vi "find_correction.vi"(9 "T1_parameters":T1, 10 "triggers":u32[][](array[numeric]), 11 "detections":u32[](array[numeric])) -> (3 "shift_us":dbl)   [LabVIEW 2014]
uses:
  <vilib>/Analysis/3filter.llb/FIR Filter (DBL).vi
  <vilib>/Analysis/NI_AALPro.lvlib
  <vilib>/Analysis/NI_AALBase.lvlib
panel:
  out "pulses":u32[](graph)
  out "derivative":dbl[](graph)
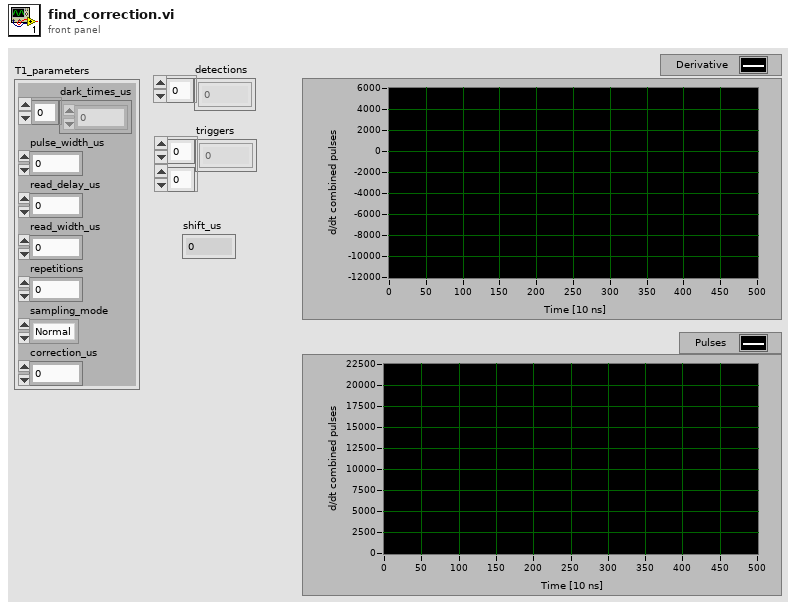
[diagram p1: front panel]
types:
  T1 = cluster{"dark_times_us":dbl[], "pulse_width_us":dbl, "read_delay_us":dbl, "read_width_us":dbl, "repetitions":i32, "sampling_mode":enum16{"Normal", "Sweep"}, "correction_us":dbl}
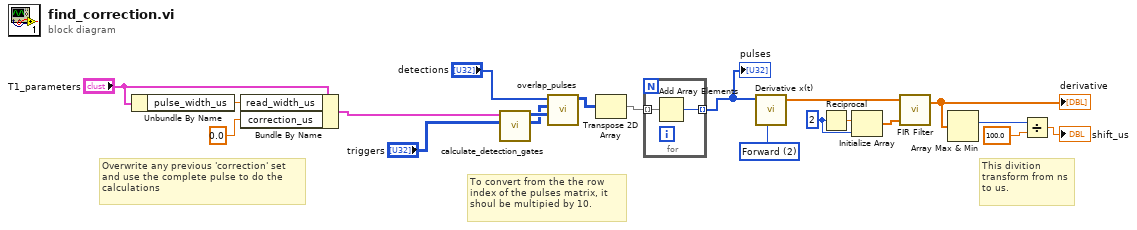
[diagram p0: block diagram]
diagram:
  w4 = 2 ("dimension size")
  w19 = u16 2 items=["2nd Order Central", "4th Order Central", "Forward", "Backward"] ("method")
  # "Overwrite any previous 'correction' set\nand use the complete pulse to do the\ncalculations"
  # "This divition transform from ns to us."
  # "To convert from the the row index of the pulses matrix, it shoul be multipied by 10."
  n1 = Unbundle By Name("T1_parameters") -> ("pulse_width_us"=w15:dbl)
  n2 = Bundle By Name(cluster="T1_parameters", "read_width_us"=w15, "correction_us"=0.0) -> (w7:T1)
  n3 = call "calculate_detection_gates.vi"("triggers"="triggers", "T1_parameters"=w7) -> ("start_read"=w11:u32[][], "stop_read"=w13:u32[][])  [unwired: 8 in]
  n4 = call "overlap_pulses.vi"("stop_read"=w13, "start_read"=w11, "detections"="detections") -> ("pulses"=w12:u32[][])  [unwired: 8 in]
  n5 = Transpose 2D Array(2D array=w12) -> (transposed array=w20:u32[][])
  n6 = for {
    tunnel: w20 -> [w22] mode=indexing
    tunnel: [w21] -> w1 mode=indexing
    n7 = Add Array Elements(numeric array=w22) -> (sum=w21:u32)
  }
  "pulses" <- w1
  n8 = call <vilib>:"Derivative x(t).vi"("method"=w19, "X"=w1) -> ("dX/dt"=w3:dbl[])  [unwired: 8 in, 1 out]
  n9 = Reciprocal(x=w4) -> (1/x=w6:dbl)
  n10 = Initialize Array(w6, w4) -> (w5:dbl[])
  n11 = call-poly <vilib>:"FIR Filter.vi"("FIR Coefficients"=w5, "X"=w3) -> ("Filtered X"=w2:dbl[])  [unwired: 2 in, 1 out]
  "derivative" <- w2
  n12 = Array Max & Min(array=w2) -> (max index (indices)=w16:i32)  [unwired: 3 out]
  n13 = Divide(x=w16, y=100.0) -> (x/y=→"shift_us":dbl)
